vi "Send Error.vi"(8 "error in (no error)":errorcluster, 11 "Ancestor in":refnum<class "Ancestor.lvclass">) -> (0 "error out":errorcluster, 3 "Ancestor out":refnum<class "Ancestor.lvclass">)   [LabVIEW 2026, in "TALOS.lvlib" / "Ancestor.lvlib" / "Ancestor.lvclass"]
doc: "Use this VI to send an error to be processed by the Error Manager of the Distributed System.\n#What if the ASV update gives an error?"
uses:
  Ancestor.lvclass
  Classes/Circus Shared Variables/Circus Shared Variables.lvclass
  TALOS.lvlib
  Internal uServices/System uServices/Error Manager/Error Info.ctl
  Internal uServices/System uServices/Error Manager/Error Manager.lvclass
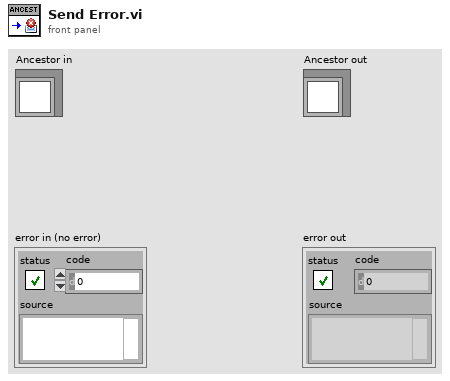
[diagram p1: front panel]
types:
  T1 = typedef "TALOS.lvlib/Error Manager.lvlib/Error Manager.lvclass/Error Info.ctl" = cluster{"error out":errorcluster, "Time Stamp":timestamp, "Machine Name":string, "GUID":string}
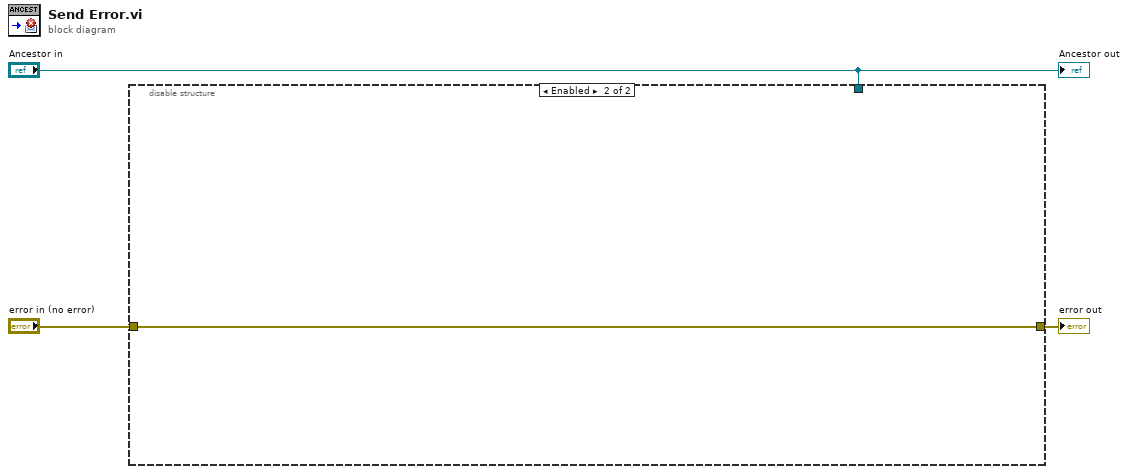
[diagram p0: block diagram]
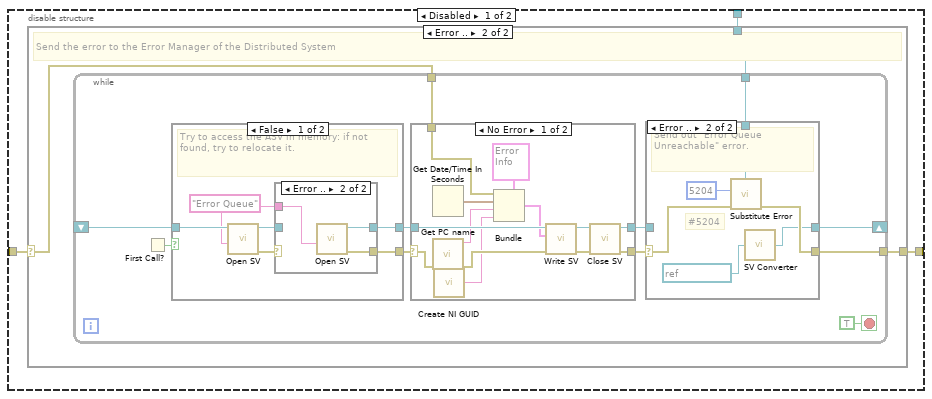
[diagram p2: hidden frame]
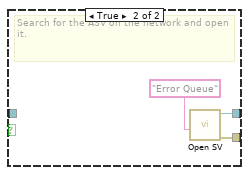
[diagram p5: hidden frame]
diagram:
  n1 = disable-structure shown="Enabled" {
    disable-tunnel: [w6 w59] -> w3
    disable-tunnel: "error in (no error)" -> [w5 w59]
    disable-tunnel: "Ancestor in" -> [w4 _]
    frame Disabled {
      n2 = case shown="Error .." w5 {
        selector: w5 -> [w7 w9]
        tunnel: [w7 w10] -> w6
        tunnel: w4 -> [_ w8]
        frame No Error {
          # "If no error, do nothing!"
        }
        frame Error {
          # "Send the error to the Error Manager of the Distributed System"
          n3 = while {
            shift-right: [w20] -> _
            shift-left: _ -> [w19]
            tunnel: [w18] -> w10
            tunnel: w9 -> [w17]
            tunnel: w8 -> [w16]
            stop <- TRUE stop-if-true
            n4 = First Call?() -> (First Call?: T/F=w11:bool)
            n5 = case shown="False" w11 {
              tunnel: [w24 w35] -> w14
              tunnel: [w23 w34] -> w13
              tunnel: w19 -> [w27 _]
              frame False {
                w22 = "Error Queue" ("SV Name")
                # "Try to access the ASV in memory: if not found, try to relocate it."
                n6 = call "Open SV.vi"("SV Name"=w22, "AEgIS Shared Variables in"=w27) -> ("error out"=w26:errorcluster, "AEgIS Shared Variables out"=w25:refnum<class "Circus Shared Variables.lvclass">)  [unwired: 8 in]
                n7 = case shown="Error .." w26 {
                  selector: w26 -> [w28 _]
                  tunnel: w25 -> [w29 _]
                  tunnel: [w29 w32] -> w24
                  tunnel: [w28 w31] -> w23
                  tunnel: w22 -> [_ w30]
                  frame No Error {
                  }
                  frame Error {
                    n8 = call "Open SV.vi"("SV Name"=w30) -> ("error out"=w31:errorcluster, "AEgIS Shared Variables out"=w32:refnum<class "Circus Shared Variables.lvclass">)  [unwired: 9 in]
                  }
                }
              }
              frame True {
                # "Search for the ASV on the network and open it."
                n9 = call "Open SV.vi"("SV Name"="Error Queue") -> ("error out"=w34:errorcluster, "AEgIS Shared Variables out"=w35:refnum<class "Circus Shared Variables.lvclass">)  [unwired: 9 in]
              }
            }
            n10 = case shown="No Error" w13 {
              selector: w13 -> [w51 w57]
              tunnel: w17 -> [w47 _]
              tunnel: [w54 w58] -> w15
              tunnel: w14 -> [w53 w58]
              tunnel: [w52 w57] -> w12
              frame No Error {
                n11 = Get Date/Time In Seconds() -> (seconds since 1Jan1904=w49:timestamp)
                n12 = call "Get PC name.vi"("error in (no error)"=w51) -> ("error out"=w50:errorcluster, "Hostname"=w48:string)  [unwired: 9 in]
                n13 = call <vilib>:"Create NI GUID.vi"() -> ("NI GUID"=w44:string)
                n14 = Bundle(cluster=T1 {"error out"={"status"=FALSE, "code"=0, "source"=""}, "Time Stamp"=timestamp(0 s since 1904-01-01), "Machine Name"="", "GUID"=""}, "error out"=w47, "Time Stamp"=w49, "Machine Name"=w48, "GUID"=w44) -> (w45:T1)
                n15 = call "Write SV.vi"("error in (no error)"=w50, "Variant"=w45, "AEgIS Shared Variables in"=w53) -> ("error out"=w56:errorcluster, "AEgIS Shared Variables out"=w55:refnum<class "Circus Shared Variables.lvclass">)  [unwired: 7 in]
                n16 = call "Close SV.vi"("error in (no error)"=w56, "AEgIS Shared Variables in"=w55) -> ("error out"=w52:errorcluster, "AEgIS Shared Variables out"=w54:refnum<class "Circus Shared Variables.lvclass">)  [unwired: 7 in, 1 out]
              }
              frame Error {
              }
            }
            n17 = case shown="Error .." w12 {
              selector: w12 -> [w36 w43]
              tunnel: w15 -> [w37 _]
              tunnel: [w37 w39] -> w20
              tunnel: [w36 w41] -> w18
              tunnel: w16 -> [_ w40]
              frame No Error {
              }
              frame Error {
                # "#5204"
                # "Send out \"Error Queue Unreachable\" error."
                n18 = call "Substitute Error.vi"("LabVIEW Object"=w40, "error in (no error)"=w43, "Error Code"=5204) -> ("error out"=w41:errorcluster)  [unwired: 8 in]
                n19 = call "SV Converter.vi"("SV"=refnum<k21> "1nv4l1d") -> ("AEgIS Shared Variables out"=w39:refnum<class "Circus Shared Variables.lvclass">)  [unwired: 4 in]
              }
            }
          }
        }
      }
    }
    frame Enabled {
    }
  }
  "error out" <- w3
  "Ancestor out" <- "Ancestor in"
